vi "Mass_2_1.vi"() -> ()   [LabVIEW 2020]
uses:
  Support/Controls/Cmd_Mouse Popup.ctl
  Support/Controls/Cmd_Var Data IO.ctl
  Support/Controls/Clst_Initialize Input.ctl
  Support/Controls/Clst_Result inspec.ctl
  Variables/Global_Cal Info.vi
  Support/Public/Polymorph/Rmv Empt Arr_2D Str.vi
  Support/Public/Polymorph/Table Initialize_Str.vi
  <vilib>/express/express arith-compare/Formula/XNode/ExpressFormulaBlockNode.xnode
panel:
  out "등급":string
  in  "시험분동 추가":i32(listbox)=24
  in  "시험분동":i32(listbox)=-1
  in  "일괄변경":bool=TRUE
  in  "분동등급":string(combo)
  out "적용?":bool
  in  "다음 버튼":bool
  in  "이전 버튼":bool
  in  "제거":bool
  in  "적용":bool
  out "추가명목값":string caption="명목값"
  in  "추가":bool
  in  "추가문자열":string
  out "분해능":string caption="저울분해능 (g)"
  out "Data Out":string[][](table)
  out "단위":string
  out "호칭질량":string
  in  "기기번호":string
  out "명목값":string
  in  "편심오차":string[][](table) caption="4. 저울 편심오차 시험"
  in  "측정횟수":u32(ring)=5 items=["5회"=5, "10회"=10]
  in  "시험분동밀도":string="8000" caption="분동밀도 (kg/㎥)"
  out "감도분동":string
  out "X=S-T":string[][](table)
  out "공기밀도":string caption="공기밀도 (kg/㎥)"
  out "Header2":string[][](table)
  in  "Measured":string[][](table) caption="3. 저울 지시값"
  out "Weight info":string[][](table) caption="2. 분동식별표기"
  out "Spec":string[][](table)
  in  "Spec 변경":bool
  out "제목":string
  out "에러 출력":errorcluster
  out "Condition":string[][](table)
  out "Atm Env":string[][](table) caption="1. 측정환경"
  out "Load?":bool
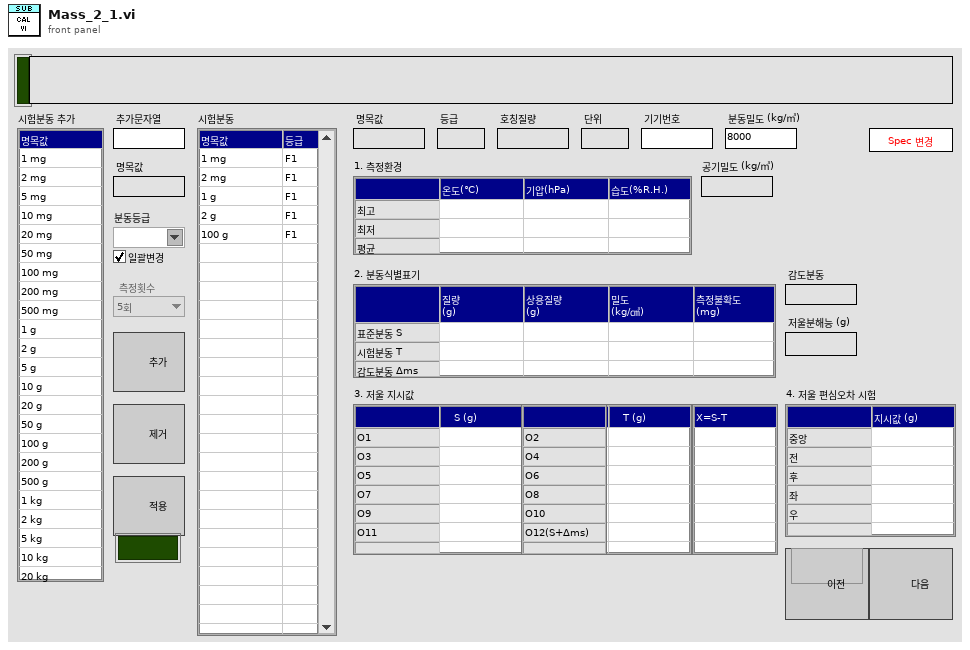
[diagram p1: front panel]
types:
  T1 = typedef "Cmd_Mouse Popup.ctl" = enum16{"활성화", "메뉴선택"}
  T2 = cluster{"Shift":bool, "Ctrl":bool, "Alt":bool, "Cmd":bool, "Opt":bool}
  T3 = typedef "Cmd_Var Data IO.ctl" = enum16{"Condition", "Condition Default", "Condition_Temp", "Resolution", "Resolution Default", "Resolution Old", "Spec", "Spec Default", "Spec Old", "Spec Temp", "Result", "Result2", "Result3", "Result_Temp", "Result_ADJ", "Result_ADJ2", "STD1", "STD2", "STD3", "STD4", "STD5", "STD Temp", "CMC", "CMC Default"}
  T4 = enum8{"Enabled", "Disabled", "Disabled and Grayed Out"}
  T5 = typedef "Clst_Initialize Input.ctl" = cluster{"Initialize 1":cluster{"Condition":refnum<vi>[], "Spec":refnum<vi>[], "Measured":refnum<vi>[], "Resolution":refnum<vi>[], "Func_ext":string, "제목":refnum<vi>, "Measured_ADJ":refnum<vi>[]}, "Initialize 2":cluster{"문자열":refnum<vi>[], "콤보박스":refnum<vi>[], "링":refnum<vi>[], "열거형":refnum<vi>[], "테이블":refnum<vi>[], "여러열":refnum<vi>[], "디지털(DBL)":refnum<vi>[], "3D string":refnum<vi>[], "ctrl":refnum<vi>[], "boolean":refnum<vi>[]}}
  T6 = typedef "Clst_Result inspec.ctl" = cluster{"분해능":string, "문자열 1":string, "문자열 2":string, "숫자형 1":i32, "숫자형 2":i32, "숫자형 3":dbl, "문자배열 1D":string[], "문자배열 2D":string[][], "문자배열 3D":string[][][], "문자배열 4D":string[][][][], "불리언 1D":bool[]}
  T7 = typedef "Clst_Atm Info Global.ctl" = cluster{"교정장소":enum16{"0 : 고정표준실", "1 : 현장교정"}, "최저온도(℃)":string, "최고온도(℃)":string, "최저습도(％ R.H.)":string, "최고습도(％ R.H.)":string, "최저기압(hPa)":string, "최고기압(hPa)":string, "교정실명":string}
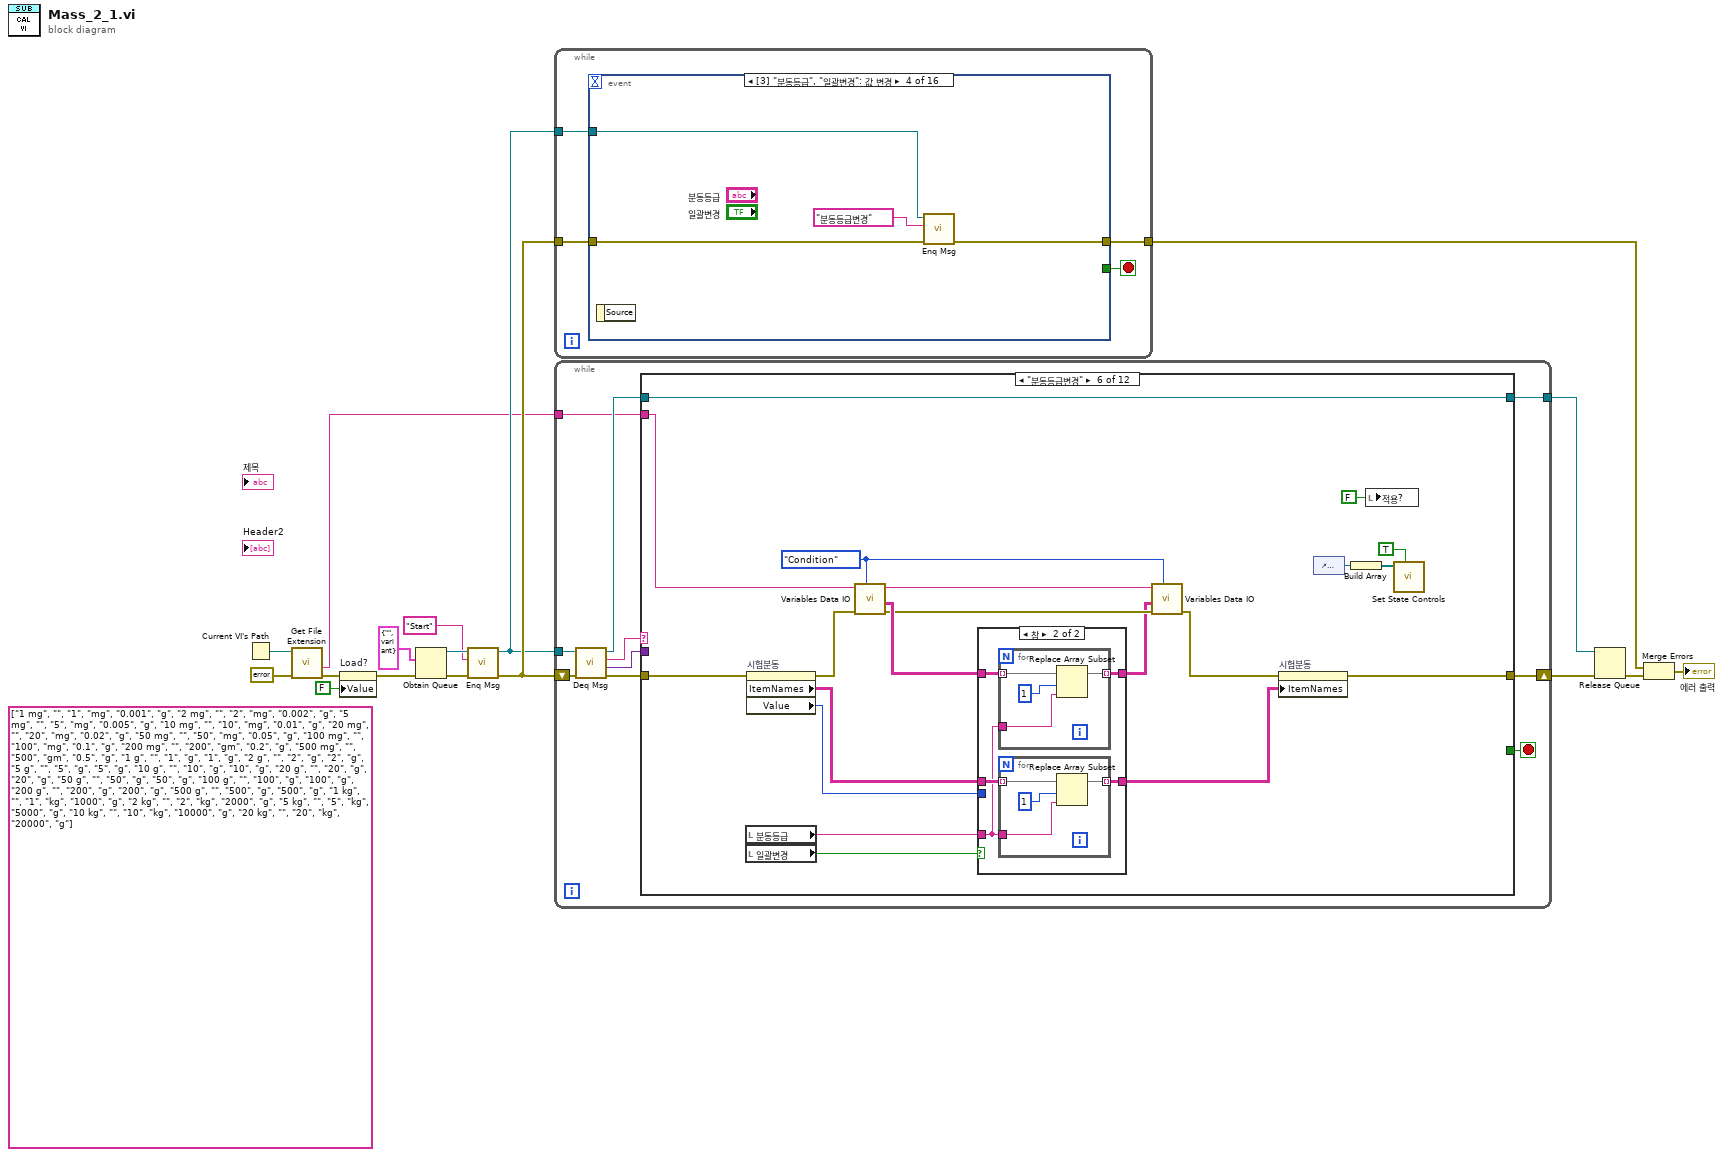
[diagram p0: block diagram]
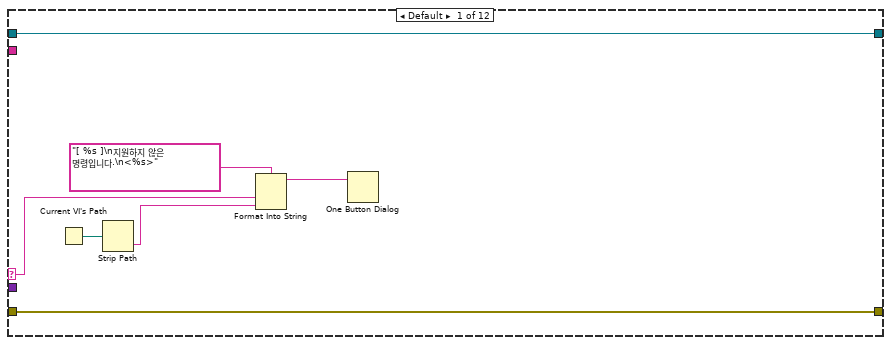
[diagram p2: hidden frame]
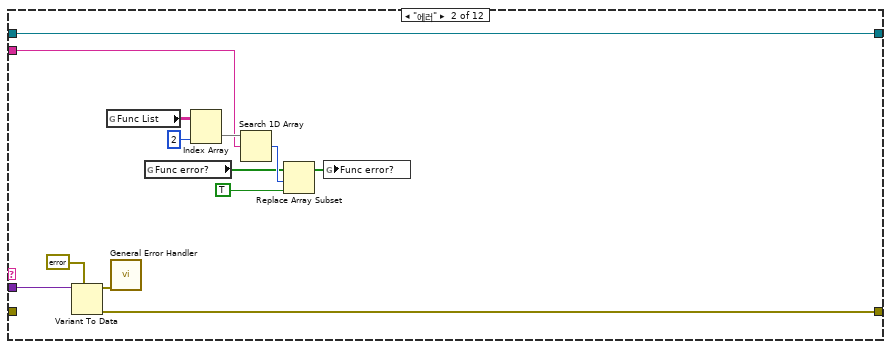
[diagram p3: hidden frame]
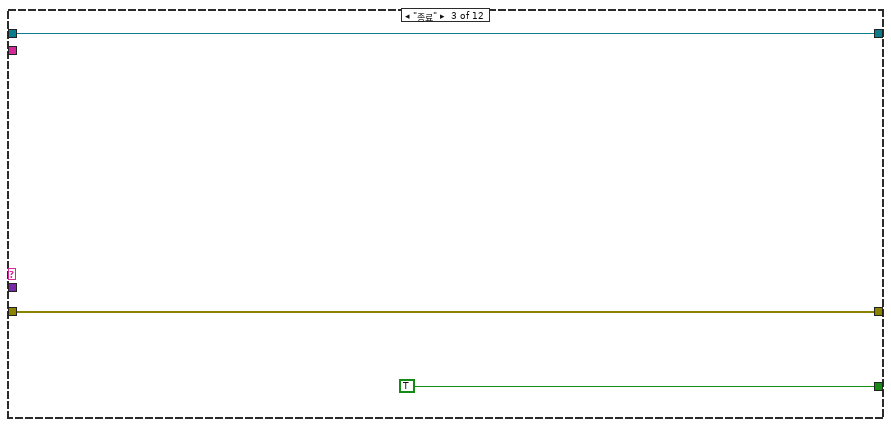
[diagram p4: hidden frame]
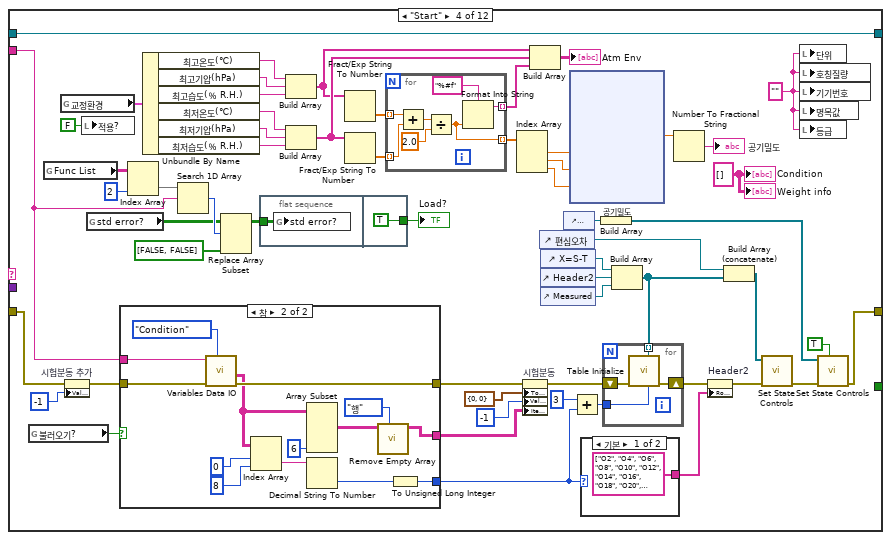
[diagram p5: hidden frame]
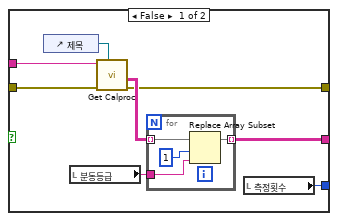
[diagram p6: hidden frame]
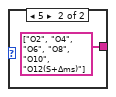
[diagram p7: hidden frame]
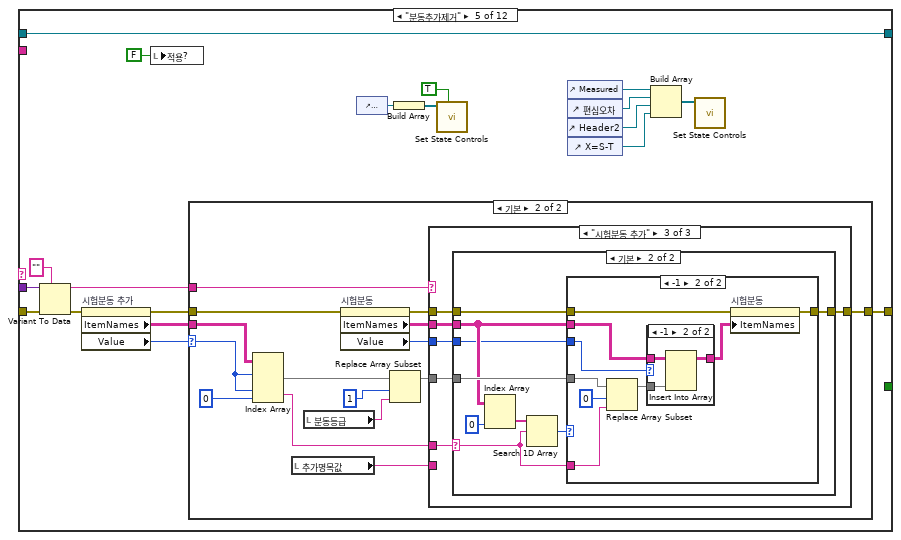
[diagram p8: hidden frame]
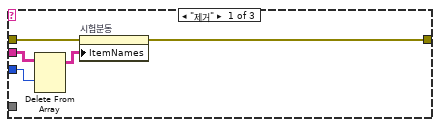
[diagram p10: hidden frame]
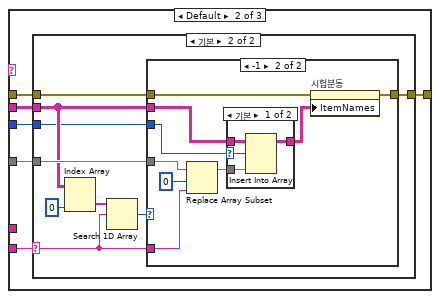
[diagram p11: hidden frame]
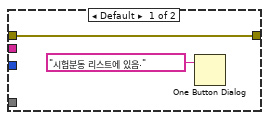
[diagram p13: hidden frame]
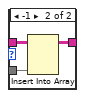
[diagram p14: hidden frame]
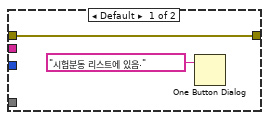
[diagram p16: hidden frame]
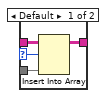
[diagram p17: hidden frame]
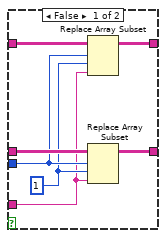
[diagram p18: hidden frame]
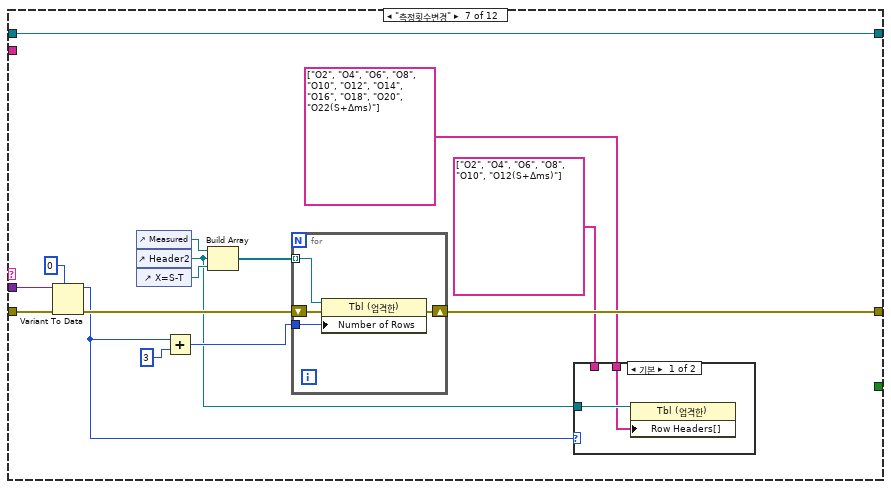
[diagram p19: hidden frame]
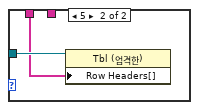
[diagram p20: hidden frame]
diagram:
  (unwired) string[][] [["1 mg", "", "1", "mg", "0.001", "g"], ["2 mg", "", "2", "mg", "0.002", "g"], ["5 mg", "", "5", "mg", "0.005", "g"], ["10 mg", "", "10", "mg", "0.01", "g"], ["20 mg", "", "20", "mg", "0.02", "g"], ["50 mg", "", "50", "mg", "0.05", "g"], ["100 mg", "", "100", "mg", "0.1", "g"], ["200 mg", "", "200", "gm", "0.2", "g"], ["500 mg", "", "500", "gm", "0.5", "g"], ["1 g", "", "1", "g", "1", "g"], ["2 g", "", "2", "g", "2", "g"], ["5 g", "", "5", "g", "5", "g"], ["10 g", "", "10", "g", "10", "g"], ["20 g", "", "20", "g", "20", "g"], ["50 g", "", "50", "g", "50", "g"], ["100 g", "", "100", "g", "100", "g"], ["200 g", "", "200", "g", "200", "g"], ["500 g", "", "500", "g", "500", "g"], ["1 kg", "", "1", "kg", "1000", "g"], ["2 kg", "", "2", "kg", "2000", "g"], ["5 kg", "", "5", "kg", "5000", "g"], ["10 kg", "", "10", "kg", "10000", "g"], ["20 kg", "", "20", "kg", "20000", "g"]] ("배열")
  n1 = Current VI's Path() -> (path=w5:path)
  n2 = call <vilib>:"Get File Extension.vi"("error in (no error)"=errorcluster {"status"=FALSE, "code"=0, "source"=""} ("에러 상수"), "file"=w5) -> ("error out"=w3:errorcluster, "filename without extension"=w4:string)  [unwired: 5 in, 3 out]
  n3 = property on="Load?" class="Bool (엄격한)"(error in=w3, "Value"=FALSE ("Load?")) -> (error out=w2:errorcluster)  [unwired: 1 in, 1 out]
  n4 = Obtain Queue(element data type=cluster{"메세지":string, "값":variant} {"메세지"="", "값"=variant} ("Message Cluster"), error in (no error)=w2) -> (queue out=w14:refnum<queue>, error out=w16:errorcluster)  [unwired: 3 in, 1 out]
  n5 = call "Enq Msg.vi"("에러 입력(에러 없음)"=w16, "메세지"="Start", "큐 입력"=w14) -> ("에러 출력"=w15:errorcluster, "큐 출력"=w12:refnum<queue>)  [unwired: 7 in]
  n6 = while {
    tunnel: w15 -> [w19]
    tunnel: w12 -> [w20]
    tunnel: [w18] -> w9
    stop <- w21 stop-if-true
    n7 = event shown="[3] \"분동등급\", \"일괄변경\": 값 변경" {
      selector: _ -> [_ _ _ _ _ _ _ _ _ _ _ _ _ _ _ _]
      dyn-events: _ -> [_ _ _ _ _ _ _ _ _ _ _ _ _ _ _ _]
      timeout: _ -> [_ _ _ _ _ _ _ _ _ _ _ _ _ _ _ _]
      tunnel: [w26 _ _ _ _ _ _ _ _ _ _ _ _ _ _ _] -> w21
      tunnel: w20 -> [w24 _ w41 w50 w55 w66 w81 w90 _ w111 w124 _ w131 _ w144 w160]
      tunnel: w19 -> [w25 w34 w48 w49 w57 w64 w83 w92 w104 w113 w125 w128 w136 w143 w146 w154]
      tunnel: [w22 w29 w40 w51 w56 w65 w82 w86 w104 w112 w123 w127 w130 w142 w145 w162] -> w18
      event Panel Close? {
        w26 = TRUE ("버림?")
        n8 = event-data() -> ()  [unwired: 1 in, 1 out]
        n9 = call "Enq Msg.vi"("에러 입력(에러 없음)"=w25, "메세지"="종료", "큐 입력"=w24) -> ("에러 출력"=w22:errorcluster)  [unwired: 7 in, 1 out]
        n10 = event-data("Discard?"=w26) -> ()  [unwired: 1 in, 1 out]
      }
      event "시험분동 추가", "추가문자열": Value Change {
        n11 = event-data() -> ()  [unwired: 1 in, 1 out]
        n12 = property on="시험분동 추가" class="MCListbox (엄격한)"(error in=w34) -> (error out=w29:errorcluster, "ItemNames"=w33:string[][])  [unwired: 1 in, 1 out]
        n13 = Index Array(array=w33, index (row) #1="시험분동 추가", index (row) #2="시험분동 추가", index (col) #2=0 ("비활성화된 인덱스 (열)")) -> (element #2=w30:string)  [unwired: 1 in, 1 out]
        n14 = case shown="기본" "추가문자열" {
          selector: "추가문자열" -> [_ w36]
          tunnel: w30 -> [w35 w38]
          tunnel: [w35 w37] -> w28
          frame "" {
          }
          frame Default {
            n15 = Format Into String(format string="%s (%s)" ("포맷 문자열"), w38, w36) -> (resulting string=w37:string)  [unwired: 2 in, 1 out]
          }
        }
        "추가명목값" <- w28
      }
      event "추가", "제거": Value Change; "시험분동 추가": Double Click {
        n16 = event-data() -> ("CtlRef"=w47:refnum<vi>)  [unwired: 1 in]
        n17 = property class="Ctl"(reference=w47, error in=w48) -> (error out=w43:errorcluster, "Label.Text"=w42:string)  [unwired: 1 out]
        n18 = To Variant(anything=w42) -> (Variant=w44:variant)
        n19 = call "Enq Msg.vi"("에러 입력(에러 없음)"=w43, "값"=w44, "메세지"="분동추가제거", "큐 입력"=w41) -> ("에러 출력"=w40:errorcluster)  [unwired: 6 in, 1 out]
        "적용?" <- FALSE ("적용?")
      }
      event "분동등급", "일괄변경": Value Change {
        n20 = event-data() -> ()  [unwired: 1 in, 1 out]
        n21 = call "Enq Msg.vi"("에러 입력(에러 없음)"=w49, "메세지"="분동등급변경", "큐 입력"=w50) -> ("에러 출력"=w51:errorcluster)  [unwired: 7 in, 1 out]
      }
      event "측정횟수": Value Change {
        n22 = event-data() -> ()  [unwired: 1 in, 1 out]
        n23 = To Variant(anything="측정횟수") -> (Variant=w54:variant)
        n24 = call "Enq Msg.vi"("에러 입력(에러 없음)"=w57, "값"=w54, "메세지"="측정횟수변경", "큐 입력"=w55) -> ("에러 출력"=w56:errorcluster)  [unwired: 6 in, 1 out]
      }
      event "적용": Value Change {
        n25 = event-data() -> ()  [unwired: 1 in, 1 out]
        n26 = property on="시험분동" class="MCListbox (엄격한)"(error in=w64) -> (error out=w63:errorcluster, "ItemNames"=w62:string[][])  [unwired: 1 in, 1 out]
        n27 = for {
          tunnel: w62 -> [w71] mode=indexing
          tunnel: [w69] -> w60 mode=indexing
          tunnel: 1 ("인덱스") -> [w67]
          n28 = Index Array(array=w71, index=w67) -> (element=w70:string)
          n29 = call <vilib>:"Trim Whitespace.vi"("string"=w70) -> ("trimmed string"=w68:string)  [unwired: 1 in]
          n30 = Empty String/Path?(string/path=w68) -> (empty?=w69:bool)
        }
        n31 = Or Array Elements(Boolean array=w60) -> (logical OR=w59:bool)
        n32 = case shown="거짓" w59 {
          tunnel: w66 -> [w78 _]
          tunnel: [w77 w80] -> w65
          tunnel: w63 -> [w76 w80]
          frame False {
            n33 = local write "적용?"(TRUE ("적용?")) -> ()
            n34 = property on="시험분동" class="MCListbox (엄격한)"(error in=w76, "Value"=-1 ("시험분동")) -> (error out=w74:errorcluster)  [unwired: 1 in, 1 out]
            n35 = call "Enq Msg.vi"("에러 입력(에러 없음)"=w74, "메세지"="Initialize", "큐 입력"=w78) -> ("에러 출력"=w77:errorcluster)  [unwired: 7 in, 1 out]
          }
          frame True {
            n36 = One Button Dialog(message="분동 등급 설정 !!!" ("메시지")) -> ()  [unwired: 1 in, 1 out]
          }
        }
      }
      event "기기번호", "시험분동밀도": Value Change {
        n37 = event-data() -> ()  [unwired: 1 in, 3 out]
        n38 = call "Enq Msg.vi"("에러 입력(에러 없음)"=w83, "메세지"="분동정보변경", "큐 입력"=w81) -> ("에러 출력"=w82:errorcluster)  [unwired: 7 in, 1 out]
      }
      event "시험분동": Value Change {
        n39 = event-data() -> ()  [unwired: 1 in, 1 out]
        n40 = local read "적용?"() -> (w89:bool)
        n41 = To Variant(anything="시험분동") -> (Variant=w91:variant)
        n42 = Less Than 0?(x="시험분동") -> (x < 0?=w85:bool)
        n43 = case shown="거짓" w89 {
          tunnel: w92 -> [w98 w102]
          tunnel: [w98 w101] -> w87
          tunnel: w91 -> [_ w100]
          tunnel: w90 -> [_ w99]
          frame False {
            n44 = control-ref of="Measured"() -> (w94:refnum<vi>)
            n45 = control-ref of="편심오차"() -> (w93:refnum<vi>)
            n46 = control-ref of="Header2"() -> (w96:refnum<vi>)
            n47 = control-ref of="X=S-T"() -> (w97:refnum<vi>)
            n48 = Build Array(w94, w93, w96, w97) -> (w95:refnum<vi>[])
            n49 = call "Set State Controls.vi"("컨트롤 참조 배열 in"=w95) -> ()  [unwired: 9 in, 2 out]
          }
          frame True {
            n50 = call "Enq Msg.vi"("에러 입력(에러 없음)"=w102, "값"=w100, "메세지"="시험분동선택", "큐 입력"=w99) -> ("에러 출력"=w101:errorcluster)  [unwired: 6 in, 1 out]
          }
        }
        n51 = property on="일괄변경" class="Bool (엄격한)"(error in=w87, "Value"=w85) -> (error out=w86:errorcluster)  [unwired: 1 in, 1 out]
      }
      event "시험분동": Drag Ended {
        n52 = event-data() -> ()  [unwired: 1 in, 4 out]
        n53 = control-ref of="Measured"() -> (w106:refnum<vi>)
        n54 = control-ref of="편심오차"() -> (w105:refnum<vi>)
        n55 = control-ref of="Header2"() -> (w108:refnum<vi>)
        n56 = control-ref of="X=S-T"() -> (w109:refnum<vi>)
        n57 = local write "적용?"(FALSE ("적용?")) -> ()
        n58 = Build Array(w106, w105, w108, w109) -> (w107:refnum<vi>[])
        n59 = call "Set State Controls.vi"("컨트롤 참조 배열 in"=w107) -> ()  [unwired: 9 in, 2 out]
      }
      event "시험분동": Double Click {
        n60 = event-data() -> ()  [unwired: 1 in, 1 out]
        n61 = local read "적용?"() -> (w114:bool)
        n62 = case shown="거짓" w114 {
          tunnel: w113 -> [w116 w121]
          tunnel: [w118 w121] -> w112
          tunnel: w111 -> [w117 _]
          frame False {
            n63 = To Variant(anything="제거") -> (Variant=w119:variant)
            n64 = call "Enq Msg.vi"("에러 입력(에러 없음)"=w116, "값"=w119, "메세지"="분동추가제거", "큐 입력"=w117) -> ("에러 출력"=w118:errorcluster)  [unwired: 6 in, 1 out]
          }
          frame True {
          }
        }
      }
      event "Measured", "편심오차": Value Change {
        n65 = event-data() -> ()  [unwired: 1 in, 3 out]
        n66 = call "Enq Msg.vi"("에러 입력(에러 없음)"=w125, "메세지"="Value Change", "큐 입력"=w124) -> ("에러 출력"=w123:errorcluster)  [unwired: 7 in, 1 out]
      }
      event "Measured", "편심오차": Shortcut Menu Activation? {
        n67 = event-data() -> ("MenuRef"=w126:refnum<k9>)  [unwired: 1 in]
        n68 = call "Mouse PopUp Control.vi"("type"=Cmd_Mouse_Popup."활성화", "error in"=w128, "메뉴 참조"=w126) -> ("error out"=w127:errorcluster)  [unwired: 8 in]
        n69 = event-data() -> ()  [unwired: 2 in, 1 out]
      }
      event "Measured", "편심오차": Shortcut Menu Selection (User) {
        n70 = event-data() -> ("CtlRef"=w134:refnum<vi>, "ItemTag"=w135:string)  [unwired: 1 in]
        n71 = call "Mouse PopUp Control.vi"("type"=Cmd_Mouse_Popup."메뉴선택", "error in"=w136, "아이템 태그"=w135, "Tbl 참조 번호"=w134) -> ("error out"=w132:errorcluster)  [unwired: 7 in]
        n72 = call "Enq Msg.vi"("에러 입력(에러 없음)"=w132, "메세지"="Value Change", "큐 입력"=w131) -> ("에러 출력"=w130:errorcluster)  [unwired: 7 in, 1 out]
      }
      event "Measured", "편심오차", "Condition": Key Down; "Measured", "편심오차", "Condition": Key Repeat {
        n73 = event-data() -> ("PlatMods"=w138:T2, "ScanCode"=w141:i16, "Mods.Num Pad"=w140:bool, "CtlRef"=w139:refnum<vi>)  [unwired: 1 in]
        n74 = call "Cursor Control.vi"("플랫폼 조합키"=w138, "참조"=w139, "Num Pad"=w140, "ScanCode"=w141, "error in"=w143) -> ("error out"=w142:errorcluster)  [unwired: 5 in, 1 out]
      }
      event "Spec 변경": Value Change {
        n75 = event-data() -> ()  [unwired: 1 in, 1 out]
        n76 = call "Enq Msg.vi"("에러 입력(에러 없음)"=w146, "메세지"="Spec 변경", "큐 입력"=w144) -> ("에러 출력"=w145:errorcluster)  [unwired: 7 in, 1 out]
      }
      event "이전 버튼", "다음 버튼": Value Change {
        n77 = event-data() -> ()  [unwired: 1 in, 1 out]
        n78 = property on="시험분동" class="MCListbox (엄격한)"(error in=w154) -> (error out=w153:errorcluster, "Value"=w152:i32, "ItemNames"=w151:string[][])  [unwired: 1 in, 1 out]
        n79 = Build Array("이전 버튼", "다음 버튼") -> (w157:bool[])
        n80 = Array Size(array=w151) -> (size(s)=w150:i32[])
        n81 = Boolean Array To Number(Boolean array=w157) -> (number=w156:u32)
        n82 = Index Array(array=w150) -> (element=w149:i32)  [unwired: 1 in]
        n83 = Decrement(x=w149) -> (x-1=w148:i32)
        n84 = case shown="2" w156 {
          tunnel: w152 -> [w164 w168 w174]
          tunnel: [w164 w165 w173] -> w155
          tunnel: w148 -> [_ _ w171]
          frame Default {
          }
          frame 1 {
            n85 = Less Or Equal To 0?(x=w168) -> (x <= 0?=w169:bool)
            n86 = Decrement(x=w168) -> (x-1=w167:i32)
            n87 = Select(t=0, s=w169, f=w167) -> (s? t:f=w165:i32)
          }
          frame 2 {
            n88 = Increment(x=w174) -> (x+1=w172:i32)
            n89 = Less Or Equal?(x=w172, y=w171) -> (x <= y?=w170:bool)
            n90 = Select(t=w172, s=w170, f=w174) -> (s? t:f=w173:i32)
          }
        }
        n91 = local write "시험분동"(w155) -> ()
        n92 = To Variant(anything=w155) -> (Variant=w161:variant)
        n93 = call "Enq Msg.vi"("에러 입력(에러 없음)"=w153, "값"=w161, "메세지"="시험분동선택", "큐 입력"=w160) -> ("에러 출력"=w162:errorcluster)  [unwired: 6 in, 1 out]
      }
    }
  }
  n94 = while {
    shift-right: [w184] -> w11
    shift-left: w15 -> [w183]
    tunnel: w12 -> [w181]
    tunnel: [w176] -> w10
    tunnel: w4 -> [w175]
    stop <- w177 stop-if-true
    n95 = call "Deq Msg.vi"("에러 입력(에러 없음)"=w183, "큐 입력"=w181) -> ("에러 출력"=w182:errorcluster, "값"=w178:variant, "메세지"=w180:string, "큐 출력"=w179:refnum<queue>)  [unwired: 6 in]
    n96 = case shown="\"분동등급변경\"" w180 {
      selector: w180 -> [w187 _ _ _ _ _ _ _ _ _ _ _]
      tunnel: w182 -> [w191 _ w207 w218 w330 w442 w474 w498 w533 w628 w653 w690]
      tunnel: [w191 w201 w207 w232 w331 w444 w477 w494 w532 w583 w664 w694] -> w184
      tunnel: w179 -> [w190 w200 w205 w265 w337 w446 w481 w510 w529 w582 w668 w696]
      tunnel: w178 -> [_ w202 _ _ w329 _ w475 _ _ w627 _ _]
      tunnel: [_ _ TRUE ("버림?") _ _ _ _ _ _ _ _ _] -> w177
      tunnel: [w190 w200 w205 w265 w337 w446 w481 w510 w529 w582 w668 w696] -> w176
      tunnel: w175 -> [_ w192 _ w222 _ w434 _ w490 w531 w610 w651 w672]
      frame Default {
        n97 = Current VI's Path() -> (path=w186:path)
        n98 = Strip Path(path=w186) -> (name=w185:string)  [unwired: 1 out]
        n99 = Format Into String(format string="[ %s ]\n지원하지 않은 명령입니다.\n<%s>" ("메시지"), w187, w185) -> (resulting string=w188:string)  [unwired: 2 in, 1 out]
        n100 = One Button Dialog(message=w188) -> ()  [unwired: 1 in, 1 out]
      }
      frame "에러" {
        n101 = Variant To Data(type=errorcluster {"status"=FALSE, "code"=0, "source"=""} ("에러 출력"), Variant=w202) -> (data=w204:errorcluster, error out=w201:errorcluster)  [unwired: 1 in]
        n102 = global read "Global_Cal Info.vi" "Func List"() -> (w194:string[][])
        n103 = call <vilib>:"General Error Handler.vi"("error in (no error)"=w204) -> ()  [unwired: 10 in, 5 out]
        n104 = global read "Global_Cal Info.vi" "Func error?"() -> (w197:bool[])
        n105 = Index Array(array=w194, index (col)=2 ("비활성화된 인덱스 (열)")) -> (element=w195:string[])  [unwired: 1 in]
        n106 = Search 1D Array(1D array=w195, element=w192) -> (index of element=w198:i32)  [unwired: 1 in]
        n107 = Replace Array Subset(array=w197, new element=TRUE ("새 원소/부분배열"), index=w198) -> (w199:bool[])
        n108 = global write "Global_Cal Info.vi" "Func error?"(w199) -> ()
      }
      frame "종료" {
      }
      frame "Start" {
        w233 = "" ("기기번호")
        w231 = string[][] []
        n109 = global read "Global_Cal Info.vi" "불러오기?"() -> (w219:bool)
        n110 = global read "Global_Cal Info.vi" "Func List"() -> (w224:string[][])
        n111 = global read "Global_Cal Info.vi" "교정환경"() -> (w240:T7)
        n112 = property on="시험분동 추가" class="MCListbox (엄격한)"(error in=w218, "Value"=-1 ("값")) -> (error out=w217:errorcluster)  [unwired: 1 in, 1 out]
        n113 = local write "적용?"(FALSE ("적용?")) -> ()
        n114 = global read "Global_Cal Info.vi" "std error?"() -> (w226:bool[][])
        n115 = case shown="참" w219 {
          tunnel: [w272 w281] -> w215
          tunnel: w222 -> [w269 w290]
          tunnel: w217 -> [w268 w291]
          tunnel: [w267 w288] -> w212
          tunnel: [w266 w279] -> w211
          frame False {
            n116 = control-ref of="제목"() -> (w273:refnum<vi>)
            n117 = local read "분동등급"() -> (w271:string)
            n118 = call "Get Calproc.vi"("제목"=w273, "에러 입력"=w268, "Func_ext"=w269) -> ("에러 출력"=w267:errorcluster, "Condition"=w270:string[][])  [unwired: 5 in, 2 out]
            n119 = for {
              tunnel: w270 -> [w277] mode=indexing
              tunnel: w271 -> [w276]
              tunnel: [w275] -> w266 mode=indexing
              n120 = Replace Array Subset(array=w277, new element=w276, index=1 ("인덱스")) -> (w275:string[])
            }
            n121 = local read "측정횟수"() -> (w272:u32)
          }
          frame True {
            n122 = call "Variables Data IO.vi"("Select"=Cmd_Var_Data_IO."Condition", "error in"=w291, "Func_ext"=w290) -> ("error out"=w288:errorcluster, "Data Out"=w286:string[][])  [unwired: 6 in, 1 out]
            n123 = Index Array(array=w286, index (row)=0 ("인덱스 (행)"), index (col)=8 ("비활성화된 인덱스 (열)")) -> (element=w283:string)
            n124 = Array Subset(array=w286, length (col)=6 ("길이")) -> (w280:string[][])  [unwired: 3 in]
            n125 = Decimal String To Number(string=w283) -> (number=w282:i32)  [unwired: 2 in, 1 out]
            n126 = call-poly "Remove Empty Array.vi"("조건"=enum16{"행", "열", "행,열"}."행", "Data in"=w280) -> ("Data out"=w279:string[][])  [unwired: 8 in, 1 out]
            n127 = To Unsigned Long Integer(number=w282) -> (unsigned 32bit integer=w281:u32)
          }
        }
        n128 = Index Array(array=w224, index (col)=2 ("비활성화된 인덱스 (열)")) -> (element=w225:string[])  [unwired: 1 in]
        n129 = Unbundle By Name(w240) -> ("최고온도(℃)"=w249:string, "최고기압(hPa)"=w250:string, "최고습도(％ R.H.)"=w252:string, "최저온도(℃)"=w251:string, "최저기압(hPa)"=w241:string, "최저습도(％ R.H.)"=w242:string)
        n130 = Search 1D Array(1D array=w225, element=w222) -> (index of element=w228:i32)  [unwired: 1 in]
        n131 = Replace Array Subset(array=w226, new element=bool[] [FALSE, FALSE] ("새 원소/부분배열"), index (row)=w228) -> (w227:bool[][])  [unwired: 1 in]
        n132 = flat-sequence {
          tunnel: w227 -> [w292]
          tunnel: [TRUE ("Load?")] -> w220
          frame #0 {
            n133 = global write "Global_Cal Info.vi" "std error?"(w292) -> ()
          }
          frame #1 {
          }
        }
        n134 = Build Array(w249, w250, w252) -> (w253:string[])
        n135 = Build Array(w251, w241, w242) -> (w254:string[])
        n136 = Fract/Exp String To Number(string=w253) -> (number=w243:dbl[])  [unwired: 3 in, 1 out]
        n137 = Fract/Exp String To Number(string=w254) -> (number=w244:dbl[])  [unwired: 3 in, 1 out]
        n138 = for {
          tunnel: w243 -> [w300] mode=indexing
          tunnel: w244 -> [w299] mode=indexing
          tunnel: [w295] -> w255 mode=indexing
          tunnel: [w294] -> w245 mode=indexing
          n139 = Add(x=w300, y=w299) -> (x+y=w298:dbl)
          n140 = Divide(x=w298, y=2.0) -> (x/y=w294:dbl)
          n141 = Format Into String(format string="%#f" ("포맷 문자열"), w294) -> (resulting string=w295:string)  [unwired: 2 in, 1 out]
        }
        n142 = Index Array(array=w245) -> (element #1=w246:dbl, element #2=w247:dbl, element #3=w248:dbl)  [unwired: 3 in]
        n143 = property on="시험분동" class="MCListbox (엄격한)"(error in=w212, "TopLeft"=cluster{"Row":u32, "Column":u32} {"Row"=0, "Column"=0} ("왼쪽 위에 보이는 셀"), "Value"=-1 ("값"), "ItemNames"=w211) -> (error out=w210:errorcluster)  [unwired: 1 in, 1 out]
        n144 = Build Array(w253, w254, w255) -> (→"Atm Env":string[][])
        n145 = control-ref of="편심오차"() -> (w239:refnum<vi>)
        n146 = control-ref of="X=S-T"() -> (w264:refnum<vi>)
        n147 = control-ref of="Header2"() -> (w263:refnum<vi>)
        n148 = control-ref of="Measured"() -> (w262:refnum<vi>)
        n149 = control-ref of="측정횟수"() -> (w236:refnum<vi>)
        n150 = xnode ("공기밀도")("t"=w246, "p"=w247, "h"=w248) -> ("결과"=w256:dbl)  [unwired: 1 in, 1 out]
        n151 = Add(x=u32 3 ("y"), y=w215) -> (x+y=w213:u32)
        n152 = case shown="기본" w215 {
          tunnel: [string[] ["O2", "O4", "O6", "O8", "O10", "O12", "O14", "O16", "O18", "O20", "O22(S+Δms)"] ("행 헤더 문자열[]") string[] ["O2", "O4", "O6", "O8", "O10", "O12(S+Δms)"] ("행 헤더 문자열[]")] -> w261
          frame Default {
          }
          frame 5 {
          }
        }
        n153 = Build Array(w236) -> (w235:refnum<vi>[])
        n154 = Build Array(w264, w263, w262) -> (w259:refnum<vi>[])
        n155 = for {
          tunnel: w259 -> [w314] mode=indexing
          tunnel: w213 -> [w313]
          shift-right: [w315] -> w260
          shift-left: w210 -> [w316]
          n156 = call-poly "Table Initialize.vi"("행의 개수"=w313, "Table Ref"=w314, "에러 입력"=w316) -> ("에러 출력"=w315:errorcluster)  [unwired: 6 in, 2 out]
        }
        n157 = Number To Fractional String(number=w256) -> (F-format string=→"공기밀도":string)  [unwired: 3 in]
        n158 = property on="Header2" class="Tbl (엄격한)"(error in=w260, "Row Headers[]"=w261) -> (error out=w258:errorcluster)  [unwired: 1 in, 1 out]
        n159 = Build Array (concatenate)(w239, w259) -> (w257:refnum<vi>[])
        n160 = call "Set State Controls.vi"("error in (no error)"=w258, "컨트롤 참조 배열 in"=w257) -> ("error out"=w216:errorcluster)  [unwired: 8 in, 1 out]
        n161 = local write "단위"(w233) -> ()
        n162 = local write "호칭질량"(w233) -> ()
        n163 = local write "기기번호"(w233) -> ()
        n164 = local write "명목값"(w233) -> ()
        n165 = local write "등급"(w233) -> ()
        n166 = call "Set State Controls.vi"("활성화 (F)"=TRUE, "error in (no error)"=w216, "컨트롤 참조 배열 in"=w235) -> ("error out"=w232:errorcluster)  [unwired: 7 in, 1 out]
        "Condition" <- w231
        "Weight info" <- w231
        "Load?" <- w220
      }
      frame "분동추가제거" {
        n167 = Variant To Data(error in=w330, type="", Variant=w329) -> (data=w328:string, error out=w326:errorcluster)
        n168 = property on="시험분동 추가" class="MCListbox (엄격한)"(error in=w326) -> (error out=w325:errorcluster, "ItemNames"=w324:string[][], "Value"=w319:i32)  [unwired: 1 in, 1 out]
        n169 = local write "적용?"(FALSE ("적용?")) -> ()
        n170 = case shown="기본" w319 {
          selector: w319 -> [_ w339]
          tunnel: [w338 w349] -> w331
          tunnel: w328 -> [_ w348]
          tunnel: w325 -> [w338 w347]
          tunnel: w324 -> [_ w346]
          frame -1 {
          }
          frame Default {
            n171 = Index Array(array=w346, index (row) #1=w339, index (row) #2=w339, index (col) #2=0 ("비활성화된 인덱스 (열)")) -> (element #1=w340:string[], element #2=w345:string)  [unwired: 1 in]
            n172 = local read "추가명목값"() -> (w353:string)
            n173 = local read "분동등급"() -> (w344:string)
            n174 = property on="시험분동" class="MCListbox (엄격한)"(error in=w347) -> (error out=w351:errorcluster, "ItemNames"=w350:string[][], "Value"=w352:i32)  [unwired: 1 in, 1 out]
            n175 = Replace Array Subset(array=w340, new element=w344, index=1 ("인덱스")) -> (w342:string[])
            n176 = case shown="\"시험분동 추가\"" w348 {
              tunnel: w350 -> [w354 w364 w398]
              tunnel: w351 -> [w356 w363 w397]
              tunnel: [w355 w362 w396] -> w349
              tunnel: w352 -> [w357 w359 w393]
              tunnel: w353 -> [_ w361 _]
              tunnel: w345 -> [_ _ w395]
              tunnel: w342 -> [_ w360 w394]
              frame "제거" {
                n177 = Delete From Array(array=w354, index (row)=w357) -> (array with subset deleted=w358:string[][])  [unwired: 2 in, 1 out]
                n178 = property on="시험분동" class="MCListbox (엄격한)"(error in=w356, "ItemNames"=w358) -> (error out=w355:errorcluster)  [unwired: 1 in, 1 out]
              }
              frame Default {
                n179 = case shown="기본" w361 {
                  selector: w361 -> [_ w369]
                  tunnel: w364 -> [_ w367]
                  tunnel: w363 -> [w365 w372]
                  tunnel: [w365 w371] -> w362
                  tunnel: w360 -> [_ w368]
                  tunnel: w359 -> [_ w366]
                  frame "" {
                  }
                  frame Default {
                    n180 = Index Array(array=w367, index (col)=0 ("비활성화된 인덱스 (열)")) -> (element=w370:string[])  [unwired: 1 in]
                    n181 = Search 1D Array(1D array=w370, element=w369) -> (index of element=w373:i32)  [unwired: 1 in]
                    n182 = case shown="-1" w373 {
                      tunnel: w372 -> [w376 w380]
                      tunnel: [w376 w377] -> w371
                      tunnel: w369 -> [_ w384]
                      tunnel: w368 -> [_ w382]
                      tunnel: w367 -> [_ w381]
                      tunnel: w366 -> [_ w379]
                      frame Default {
                        n183 = One Button Dialog(message="시험분동 리스트에 있음." ("메시지")) -> ()  [unwired: 1 in, 1 out]
                      }
                      frame -1 {
                        n184 = Replace Array Subset(array=w382, new element=w384, index=0 ("인덱스")) -> (w383:string[])
                        n185 = case shown="기본" w379 {
                          selector: w379 -> [w387 _]
                          tunnel: w381 -> [w389 w392]
                          tunnel: w383 -> [w388 w391]
                          tunnel: [w386 w390] -> w378
                          frame Default {
                            n186 = Insert Into Array(array=w389, index (row)=w387, new element=w388) -> (w386:string[][])  [unwired: 1 in]
                          }
                          frame -1 {
                            n187 = Insert Into Array(array=w392, new element=w391) -> (w390:string[][])  [unwired: 2 in]
                          }
                        }
                        n188 = property on="시험분동" class="MCListbox (엄격한)"(error in=w380, "ItemNames"=w378) -> (error out=w377:errorcluster)  [unwired: 1 in, 1 out]
                      }
                    }
                  }
                }
              }
              frame "시험분동 추가" {
                n189 = case shown="기본" w395 {
                  selector: w395 -> [_ w403]
                  tunnel: w398 -> [_ w401]
                  tunnel: w397 -> [w399 w406]
                  tunnel: [w399 w405] -> w396
                  tunnel: w394 -> [_ w402]
                  tunnel: w393 -> [_ w400]
                  frame "" {
                  }
                  frame Default {
                    n190 = Index Array(array=w401, index (col)=0 ("비활성화된 인덱스 (열)")) -> (element=w404:string[])  [unwired: 1 in]
                    n191 = Search 1D Array(1D array=w404, element=w403) -> (index of element=w407:i32)  [unwired: 1 in]
                    n192 = case shown="-1" w407 {
                      tunnel: w406 -> [w410 w416]
                      tunnel: [w410 w415] -> w405
                      tunnel: w403 -> [_ w418]
                      tunnel: w402 -> [_ w417]
                      tunnel: w401 -> [_ w414]
                      tunnel: w400 -> [_ w412]
                      frame Default {
                        n193 = One Button Dialog(message="시험분동 리스트에 있음." ("메시지")) -> ()  [unwired: 1 in, 1 out]
                      }
                      frame -1 {
                        n194 = Replace Array Subset(array=w417, new element=w418, index=0 ("인덱스")) -> (w413:string[])
                        n195 = case shown="-1" w412 {
                          selector: w412 -> [w421 _]
                          tunnel: w414 -> [w423 w426]
                          tunnel: w413 -> [w422 w425]
                          tunnel: [w420 w424] -> w411
                          frame Default {
                            n196 = Insert Into Array(array=w423, index (row)=w421, new element=w422) -> (w420:string[][])  [unwired: 1 in]
                          }
                          frame -1 {
                            n197 = Insert Into Array(array=w426, new element=w425) -> (w424:string[][])  [unwired: 2 in]
                          }
                        }
                        n198 = property on="시험분동" class="MCListbox (엄격한)"(error in=w416, "ItemNames"=w411) -> (error out=w415:errorcluster)  [unwired: 1 in, 1 out]
                      }
                    }
                  }
                }
              }
            }
          }
        }
        n199 = control-ref of="측정횟수"() -> (w322:refnum<vi>)
        n200 = Build Array(w322) -> (w321:refnum<vi>[])
        n201 = call "Set State Controls.vi"("활성화 (F)"=TRUE, "컨트롤 참조 배열 in"=w321) -> ()  [unwired: 8 in, 2 out]
        n202 = control-ref of="Measured"() -> (w333:refnum<vi>)
        n203 = control-ref of="편심오차"() -> (w334:refnum<vi>)
        n204 = control-ref of="Header2"() -> (w335:refnum<vi>)
        n205 = control-ref of="X=S-T"() -> (w336:refnum<vi>)
        n206 = Build Array(w333, w334, w335, w336) -> (w332:refnum<vi>[])
        n207 = call "Set State Controls.vi"("컨트롤 참조 배열 in"=w332) -> ()  [unwired: 9 in, 2 out]
      }
      frame "분동등급변경" {
        w428 = Cmd_Var_Data_IO."Condition" ("Select")
        n208 = local read "분동등급"() -> (w445:string)
        n209 = local read "일괄변경"() -> (w440:bool)
        n210 = property on="시험분동" class="MCListbox (엄격한)"(error in=w442) -> (error out=w435:errorcluster, "ItemNames"=w433:string[][], "Value"=w441:i32)  [unwired: 1 in, 1 out]
        n211 = call "Variables Data IO.vi"("Select"=w428, "error in"=w435, "Func_ext"=w434) -> ("error out"=w431:errorcluster, "Data Out"=w432:string[][], "Func_ext Out"=w429:string)  [unwired: 6 in]
        n212 = case shown="참" w440 {
          tunnel: w433 -> [w453 w458]
          tunnel: [w452 w457] -> w443
          tunnel: w445 -> [w449 w455]
          tunnel: w441 -> [w451 _]
          tunnel: w432 -> [w448 w456]
          tunnel: [w447 w454] -> w427
          frame False {
            w450 = 1 ("인덱스")
            n213 = Replace Array Subset(array=w448, new element=w449, index (row)=w451, index (col)=w450) -> (w447:string[][])
            n214 = Replace Array Subset(array=w453, new element=w449, index (row)=w451, index (col)=w450) -> (w452:string[][])
          }
          frame True {
            n215 = for {
              tunnel: w456 -> [w462] mode=indexing
              tunnel: w455 -> [w459]
              tunnel: [w461] -> w454 mode=indexing
              n216 = Replace Array Subset(array=w462, new element=w459, index=1 ("인덱스")) -> (w461:string[])
            }
            n217 = for {
              tunnel: w458 -> [w466] mode=indexing
              tunnel: w455 -> [w463]
              tunnel: [w465] -> w457 mode=indexing
              n218 = Replace Array Subset(array=w466, new element=w463, index=1 ("인덱스")) -> (w465:string[])
            }
          }
        }
        n219 = call "Variables Data IO.vi"("Select"=w428, "error in"=w431, "Data In"=w427, "Func_ext"=w429) -> ("error out"=w430:errorcluster)  [unwired: 5 in, 2 out]
        n220 = property on="시험분동" class="MCListbox (엄격한)"(error in=w430, "ItemNames"=w443) -> (error out=w444:errorcluster)  [unwired: 1 in, 1 out]
        n221 = control-ref of="측정횟수"() -> (w438:refnum<vi>)
        n222 = Build Array(w438) -> (w437:refnum<vi>[])
        n223 = local write "적용?"(FALSE ("적용?")) -> ()
        n224 = call "Set State Controls.vi"("활성화 (F)"=TRUE, "컨트롤 참조 배열 in"=w437) -> ()  [unwired: 8 in, 2 out]
      }
      frame "측정횟수변경" {
        n225 = Variant To Data(error in=w474, type=u32 0, Variant=w475) -> (data=w470:u32, error out=w473:errorcluster)
        n226 = control-ref of="Measured"() -> (w480:refnum<vi>)
        n227 = control-ref of="Header2"() -> (w469:refnum<vi>)
        n228 = control-ref of="X=S-T"() -> (w479:refnum<vi>)
        n229 = Add(x=w470, y=u32 3) -> (x+y=w472:u32)
        n230 = Build Array(w480, w469, w479) -> (w478:refnum<vi>[])
        n231 = for {
          tunnel: w478 -> [w487] mode=indexing
          shift-right: [w488] -> w477
          shift-left: w473 -> [w489]
          tunnel: w472 -> [w486]
          n232 = property class="Tbl (엄격한)"(reference=w487, error in=w489, "Number of Rows"=w486) -> (error out=w488:errorcluster)  [unwired: 1 out]
        }
        n233 = case shown="기본" w470 {
          tunnel: w469 -> [w483 w485]
          tunnel: string[] ["O2", "O4", "O6", "O8", "O10", "O12", "O14", "O16", "O18", "O20", "O22(S+Δms)"] ("행 헤더 문자열[]") -> [w482 _]
          tunnel: string[] ["O2", "O4", "O6", "O8", "O10", "O12(S+Δms)"] ("행 헤더 문자열[]") -> [_ w484]
          frame Default {
            n234 = property class="Tbl (엄격한)"(reference=w483, "Row Headers[]"=w482) -> ()  [unwired: 1 in, 2 out]
          }
          frame 5 {
            n235 = property class="Tbl (엄격한)"(reference=w485, "Row Headers[]"=w484) -> ()  [unwired: 1 in, 2 out]
          }
        }
      }
      frame "Initialize" {
        n236 = control-ref of="제목"() -> (w513:refnum<vi>)
        n237 = control-ref of="Condition"() -> (w515:refnum<vi>)
        n238 = control-ref of="Spec"() -> (w512:refnum<vi>)
        n239 = control-ref of="시험분동"() -> (w505:refnum<vi>)
        n240 = control-ref of="시험분동밀도"() -> (w503:refnum<vi>)
        n241 = control-ref of="Measured"() -> (w506:refnum<vi>)
        n242 = control-ref of="편심오차"() -> (w507:refnum<vi>)
        n243 = control-ref of="Header2"() -> (w508:refnum<vi>)
        n244 = control-ref of="X=S-T"() -> (w509:refnum<vi>)
        n245 = control-ref of="측정횟수"() -> (w501:refnum<vi>)
        n246 = property on="측정횟수" class="Ring (엄격한)"(error in=w498, "DisabledEnum"=T4."Disabled and Grayed Out" ("비활성화")) -> (error out=w496:errorcluster)  [unwired: 1 in, 1 out]
        n247 = Build Array(w515) -> (w514:refnum<vi>[])
        n248 = Build Array(w512) -> (w511:refnum<vi>[])
        n249 = Build Array(w505) -> (w504:refnum<vi>[])
        n250 = Build Array(w503) -> (w502:refnum<vi>[])
        n251 = Build Array(w501) -> (w500:refnum<vi>[])
        n252 = Build Array(w506, w507, w508, w509) -> (w499:refnum<vi>[])
        n253 = Bundle By Name(cluster=T5 {"Initialize 1"={"Condition"=[], "Spec"=[], "Measured"=[], "Resolution"=[], "Func_ext"="", "제목"=refnum, "Measured_ADJ"=[]}, "Initialize 2"={"문자열"=[], "콤보박스"=[], "링"=[], "열거형"=[], "테이블"=[], "여러열"=[], "디지털(DBL)"=[], "3D string"=[], "ctrl"=[], "boolean"=[]}} ("입력 클러스터"), "Initialize 1.Func_ext"=w490, "Initialize 1.제목"=w513, "Initialize 1.Condition"=w514, "Initialize 1.Spec"=w511, "Initialize 2.여러열"=w504, "Initialize 2.문자열"=w502, "Initialize 2.링"=w500, "Initialize 2.테이블"=w499) -> (w516:T5)
        n254 = call "Initialize_etc.vi"("큐 입력"=w510, "error in"=w496, "입력 클러스터"=w516) -> ("error out"=w495:errorcluster)  [unwired: 6 in, 2 out]
        n255 = flat-sequence {
          tunnel: w495 -> [w523]
          tunnel: [w523] -> w494
          tunnel: [w522] -> w493
          tunnel: w490 -> [w521]
          frame #0 {
            n256 = global read "Global_Cal Info.vi" "Func List"() -> (w528:string[][])
            n257 = global read "Global_Cal Info.vi" "std error?"() -> (w525:bool[][])
            n258 = Index Array(array=w528, index (col)=2 ("비활성화된 인덱스 (열)")) -> (element=w527:string[])  [unwired: 1 in]
            n259 = Search 1D Array(1D array=w527, element=w521) -> (index of element=w524:i32)  [unwired: 1 in]
            n260 = Index Array(array=w525, index (row)=w524) -> (element=w522:bool[])  [unwired: 1 in]
          }
        }
        n261 = Or Array Elements(Boolean array=w493) -> (logical OR=w492:bool)
        n262 = case shown="참" w492 {
          tunnel: "%s\n※※※※※※※※※※※※※※※※※※※※※※※※※※※※※※※※\n\n!!! 기준기 교정값 확인 필수 !!!\n\n기준기 교정값에 빈 행이 있습니다.\n\n해당 교정점에 대해 기준기 교정이 되어있는지 확인하세요." ("포맷 문자열") -> [_ w520]
          tunnel: w490 -> [_ w518]
          frame False {
          }
          frame True {
            n263 = Format Into String(format string=w520, w518) -> (resulting string=w519:string)  [unwired: 2 in, 1 out]
            n264 = One Button Dialog(message=w519) -> ()  [unwired: 1 in, 1 out]
          }
        }
      }
      frame "분동정보변경" {
        n265 = local read "시험분동"() -> (w530:i32)
        n266 = case shown="기본" w530 {
          selector: w530 -> [_ w542]
          tunnel: w533 -> [w534 w535]
          tunnel: [w534 w552] -> w532
          tunnel: w531 -> [_ w539]
          tunnel: w529 -> [_ w551]
          frame -1 {
          }
          frame Default {
            n267 = local read "시험분동밀도"() -> (w546:string)
            n268 = local read "기기번호"() -> (w543:string)
            n269 = local read "Condition"() -> (w541:string[][])
            n270 = Replace Array Subset(array=w541, new element #1=w543, index (row) #1=w542, index (col) #1=6 ("비활성화된 인덱스 (열)"), new element #2=w546, index (row) #2=w542, index (col) #2=7 ("비활성화된 인덱스 (열)")) -> (w538:string[][])
            n271 = local write "Condition"(w538) -> ()
            n272 = call "Variables Data IO.vi"("Select"=Cmd_Var_Data_IO."Condition", "error in"=w535, "Data In"=w538, "Func_ext"=w539) -> ("error out"=w537:errorcluster)  [unwired: 5 in, 2 out]
            n273 = property on="Weight info" class="Tbl (엄격한)"(error in=w537) -> (error out=w545:errorcluster, "Value"=w549:string[][])  [unwired: 1 in, 1 out]
            n274 = Replace Array Subset(array=w549, new element=w546, index (row)=1 ("인덱스 (행)"), index (col)=2 ("비활성화된 인덱스 (열)")) -> (w544:string[][])
            n275 = property on="Weight info" class="Tbl (엄격한)"(error in=w545, "Value"=w544) -> (error out=w536:errorcluster)  [unwired: 1 in, 1 out]
            n276 = call "Enq Msg.vi"("에러 입력(에러 없음)"=w536, "메세지"="Value Change", "큐 입력"=w551) -> ("에러 출력"=w552:errorcluster)  [unwired: 7 in, 1 out]
          }
        }
      }
      frame "시험분동선택" {
        w586 = 2 ("비활성화된 인덱스 (열)")
        w593 = "" ("원소")
        w595 = 3 ("길이")
        n277 = Variant To Data(error in=w628, type=0, Variant=w627) -> (data=w585:i32, error out=w609:errorcluster)
        n278 = call "Variables Data IO.vi"("Select"=Cmd_Var_Data_IO."STD1", "error in"=w609, "Func_ext"=w610) -> ("error out"=w559:errorcluster, "Data Out"=w608:string[][], "Func_ext Out"=w558:string)  [unwired: 6 in]
        n279 = Multiply(x=w595, y=w585) -> (x*y=w594:i32)
        n280 = call "Variables Data IO.vi"("Select"=Cmd_Var_Data_IO."Result", "error in"=w559, "Func_ext"=w558) -> ("error out"=w568:errorcluster, "Data Out"=w596:string[][], "Func_ext Out"=w569:string)  [unwired: 6 in]
        n281 = Index Array(array=w608, index (row)=w585) -> (element=w607:string[])  [unwired: 1 in]
        n282 = Index Array(array=w607, index #1=3 ("인덱스")) -> (element #1=w605:string, element #2=w604:string, element #3=w603:string, element #4=→"감도분동":string, element #5=w602:string, element #6=w601:string, element #7=w600:string)  [unwired: 6 in]
        n283 = call "Variables Data IO.vi"("Select"=Cmd_Var_Data_IO."STD2", "error in"=w568, "Func_ext"=w569) -> ("error out"=w557:errorcluster, "Data Out"=w599:string[][], "Func_ext Out"=w556:string)  [unwired: 6 in]
        n284 = Delete From Array(array=w596, length=w595, index (col)=w594) -> (deleted portion=w590:string[][])  [unwired: 1 in, 1 out]
        "Data Out" <- w590
        n285 = call "Variables Data IO.vi"("Select"=Cmd_Var_Data_IO."Condition", "error in"=w557, "Func_ext"=w556) -> ("error out"=w555:errorcluster, "Data Out"=w612:string[][])  [unwired: 6 in, 1 out]
        n286 = Fract/Exp String To Number(string=w605) -> (number=w623:dbl)  [unwired: 3 in, 1 out]
        n287 = Fract/Exp String To Number(string=w604) -> (number=w622:dbl)  [unwired: 3 in, 1 out]
        n288 = Delete From Array(array=w590, index (row)=0 ("인덱스 (행)")) -> (array with subset deleted=w588:string[][])  [unwired: 2 in, 1 out]
        n289 = Index Array(array=w599, index (row)=w585, index (col)=1 ("비활성화된 인덱스 (열)")) -> (element=w570:string)
        "분해능" <- w570
        n290 = Fract/Exp String To Number(string=w602) -> (number=w618:dbl)  [unwired: 3 in, 1 out]
        n291 = Fract/Exp String To Number(string=w601) -> (number=w617:dbl)  [unwired: 3 in, 1 out]
        n292 = xnode ("참질량")("mc"=w623, "d"=w622) -> ("결과"=w621:dbl)  [unwired: 1 in, 1 out]
        n293 = xnode ("참질량 2")("mc"=w618, "d"=w617) -> ("결과"=w616:dbl)  [unwired: 1 in, 1 out]
        n294 = Index Array(array=w612, index (row)=w585) -> (element=w611:string[])  [unwired: 1 in]
        n295 = Delete From Array(array=w588, length=w586, index (col)=w586) -> (deleted portion=w563:string[][], array with subset deleted=w587:string[][])  [unwired: 1 in]
        n296 = Number To Fractional String(number=w621) -> (F-format string=w620:string)  [unwired: 3 in]
        n297 = Number To Fractional String(number=w616) -> (F-format string=w615:string)  [unwired: 3 in]
        n298 = Index Array(array=w611, index #5=6 ("인덱스")) -> (element #1=→"명목값":string, element #2=→"등급":string, element #3=→"호칭질량":string, element #4=→"단위":string, element #5=w577:string, element #6=w576:string)  [unwired: 5 in]
        n299 = local write "Measured"(w587) -> ()
        n300 = local read "분해능"() -> (w571:string)
        n301 = local read "편심오차"() -> (w565:string[][])
        n302 = Concatenate Strings(w563) -> (w562:string)
        n303 = Build Array(w620, w605, w604, w603) -> (w619:string[])
        n304 = Build Array(w615, w602, w601, w600) -> (w614:string[])
        n305 = call <vilib>:"Trim Whitespace.vi"("string"=w562) -> ("trimmed string"=w561:string)  [unwired: 1 in]
        n306 = Empty String/Path?(string/path=w561) -> (empty?=w560:bool)
        n307 = Equal?(x=w570, y=w571) -> (x = y?=w567:bool)
        n308 = Build Array(w593, w593, w576, w593) -> (w592:string[])
        n309 = And(x=w560, y=w567) -> (x .and. y?=w566:bool)
        n310 = Build Array(w619, w592, w614) -> (w574:string[][])
        n311 = local write "기기번호"(w577) -> ()
        n312 = local write "시험분동밀도"(w576) -> ()
        n313 = Select(t=w565, s=w566, f=w563) -> (s? t:f=w564:string[][])
        n314 = property on="Weight info" class="Tbl (엄격한)"(error in=w555, "Value"=w574) -> (error out=w575:errorcluster)  [unwired: 1 in, 1 out]
        n315 = local write "편심오차"(w564) -> ()
        n316 = call "Enq Msg.vi"("에러 입력(에러 없음)"=w575, "메세지"="Value Change", "큐 입력"=w582) -> ("에러 출력"=w583:errorcluster)  [unwired: 7 in, 1 out]
        "X=S-T" <- string[][] [] ("X=S-T")
      }
      frame "Value Change" {
        n317 = local read "시험분동"() -> (w661:i32)
        n318 = local read "측정횟수"() -> (w660:u32)
        n319 = local read "공기밀도"() -> (w659:string)
        n320 = call "Variables Data IO.vi"("Select"=Cmd_Var_Data_IO."Resolution", "error in"=w653, "Func_ext"=w651) -> ("error out"=w652:errorcluster, "Data Out"=w649:string[][], "Func_ext Out"=w650:string)  [unwired: 6 in]
        n321 = control-ref of="Weight info"() -> (w663:refnum<vi>)
        n322 = control-ref of="Data Out"() -> (w656:refnum<vi>)
        n323 = control-ref of="Measured"() -> (w655:refnum<vi>)
        n324 = control-ref of="편심오차"() -> (w657:refnum<vi>)
        n325 = Bundle By Name(cluster=T6 {"분해능"="", "문자열 1"="", "문자열 2"="", "숫자형 1"=0, "숫자형 2"=0, "숫자형 3"=0.0, "문자배열 1D"=[], "문자배열 2D"=[], "문자배열 3D"=[], "문자배열 4D"=[], "불리언 1D"=[]} ("입력 클러스터"), "숫자형 1"=w661, "숫자형 2"=w660, "문자열 1"=w659, "문자배열 2D"=w649) -> (w665:T6)
        n326 = Build Array(w663) -> (w667:refnum<vi>[])
        n327 = Build Array(w656, w655, w657) -> (w662:refnum<vi>[])
        n328 = call "Result inspection.vi"("입력 클러스터"=w665, "error in"=w652, "Ref. Data (excluded)"=w662, "Ref. Data (Inspection)"=w667, "Func ext"=w650) -> ("error out"=w664:errorcluster, "Data (spec 미적용)"=w658:string[][])  [unwired: 3 in, 2 out]
        n329 = local write "X=S-T"(w658) -> ()
      }
      frame "Spec 변경" {
        n330 = global read "Global_Cal Info.vi" "Func List"() -> (w677:string[][])
        n331 = global read "Global_Cal Info.vi" "Spec변경?"() -> (w673:bool[])
        n332 = call "Variables Data IO.vi"("Select"=Cmd_Var_Data_IO."Resolution", "error in"=w690, "Func_ext"=w672) -> ("error out"=w689:errorcluster, "Data Out"=w683:string[][], "Func_ext Out"=w688:string)  [unwired: 6 in]
        n333 = Index Array(array=w677, index (col)=2 ("비활성화된 인덱스 (열)")) -> (element=w675:string[])  [unwired: 1 in]
        n334 = Search 1D Array(1D array=w675, element=w672) -> (index of element=w674:i32)  [unwired: 1 in]
        n335 = Index Array(array=w673, index=w674) -> (element=w678:bool)
        n336 = local read "Condition"() -> (w670:string[][])
        n337 = Select(t=Cmd_Var_Data_IO."Spec Old" ("Select"), s=w678, f=Cmd_Var_Data_IO."Spec Default" ("Select")) -> (s? t:f=w671:T3)
        n338 = call "Variables Data IO.vi"("Select"=w671, "error in"=w689, "Func_ext"=w688) -> ("error out"=w691:errorcluster, "Data Out"=w682:string[][], "Func_ext Out"=w684:string)  [unwired: 6 in]
        n339 = for {
          tunnel: w670 -> [w702] mode=indexing
          tunnel: [w701] -> w669 mode=indexing
          n340 = Index Array(array=w702, index #2=4 ("인덱스")) -> (element #1=w700:string, element #2=w698:string, element #3=w697:string)  [unwired: 2 in]
          n341 = Build Array(w700, w698, w697) -> (w701:string[])
        }
        n342 = local read "Spec"() -> (w681:string[][])
        n343 = call "Spec Edit.vi"("Condition"=w669, "열번호(기준값)"=1 ("기준열(0)"), "Spec Value"=w681, "에러 입력(에러 없음)"=w691, "Resolution"=w683, "Spec Default"=w682, "Func_ext"=w684) -> ("에러 출력"=w695:errorcluster, "변경?"=w692:bool, "Spec Default out"=w686:string[][], "Spec 출력"=w693:string[][])  [unwired: 1 in]
        n344 = case shown="참" w692 {
          tunnel: w695 -> [w703 w711]
          tunnel: [w703 w707] -> w694
          tunnel: w693 -> [_ w709]
          tunnel: w684 -> [_ w710]
          tunnel: w686 -> [_ w705]
          frame False {
          }
          frame True {
            n345 = call "Variables Data IO.vi"("Select"=Cmd_Var_Data_IO."Spec", "error in"=w711, "Data In"=w709, "Func_ext"=w710) -> ("error out"=w708:errorcluster, "Func_ext Out"=w706:string)  [unwired: 5 in, 1 out]
            n346 = call "Variables Data IO.vi"("Select"=Cmd_Var_Data_IO."Spec Old", "error in"=w708, "Data In"=w705, "Func_ext"=w706) -> ("error out"=w707:errorcluster)  [unwired: 5 in, 2 out]
            "Spec" <- w709
          }
        }
      }
    }
  }
  n347 = Release Queue(queue=w10, error in (no error)=w11) -> (error out=w8:errorcluster)  [unwired: 1 in, 2 out]
  n348 = Merge Errors(w9, w8) -> (→"에러 출력":errorcluster)
